vi "Volume.vi"(8 "error in":errorcluster, 10 "Volume":i32, 11 "Channel":i32) -> (0 "error out":errorcluster, 3 "Current Volume":i32)   [LabVIEW 2014, in "LibSDL2_Mixer.lvlib"]
uses:
  LibSDL2_Mixer.lvlib
  LibSDL2 Wrapper/DLL/SDL2_mixer.dll
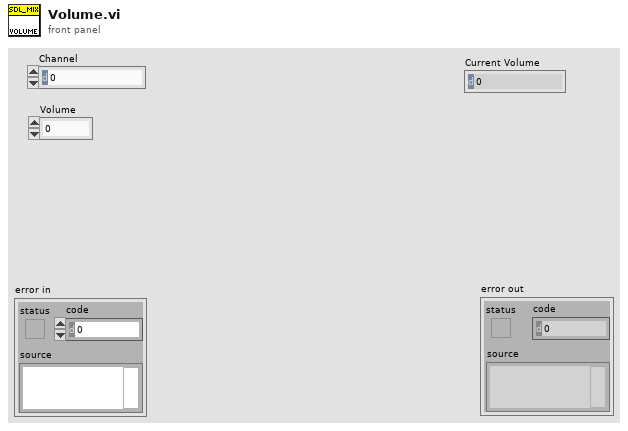
[diagram p1: front panel]
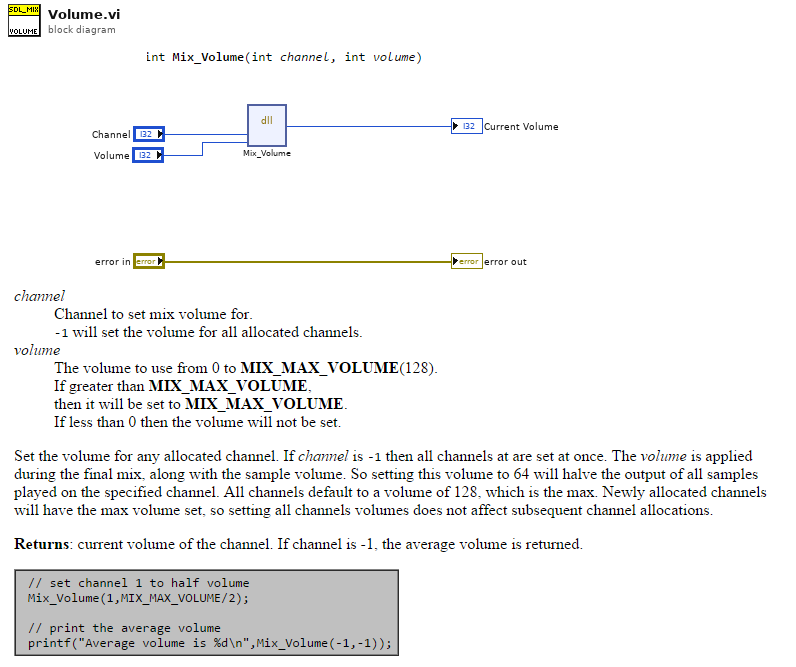
[diagram p0: block diagram]
diagram:
  n1 = dll-call lib="C:/dev/PGS/LabSDL2/Source/Libraries/LibSDL2 Wrapper/DLL/SDL2_mixer.dll" fn="Mix_Volume"("channel"="Channel", "volume"="Volume") -> ("return type"=→"Current Volume":i32)  [unwired: 5 in, 2 out]
  "error out" <- "error in"
